vi "Write DIT.vi"(5 "append to file? (default=T)":bool=TRUE, 6 "error in":errorcluster, 7 "String":string, 8 "DIT Key Info":T1, 9 "Filepath In":path) -> (0 "error out":errorcluster, 3 "Filepath Out":path)   [LabVIEW 2013]
doc: "Takes recent Activities text which has already been written to the Activities file and calculates the DIT and then appends the DIT to the Activities file.\n\nWhen this VI is used for images or other non-text file, it creates a new file with just the DIT in the attachment file. The file created has the same name as the Filepath input. Higher level VIs must determine the filename and extension."
uses:
  User Access Type defs/DIT Key cluster.ctl
  GUI/GUI.lvlib
panel:
  out "DIT":string
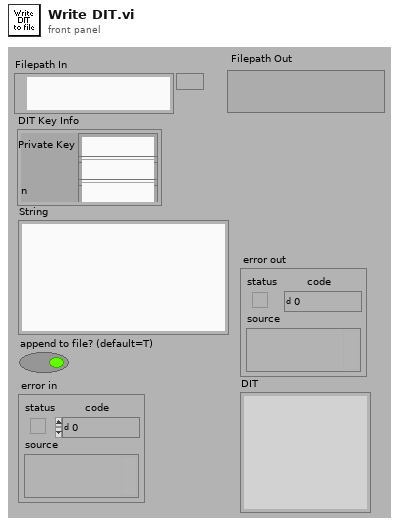
[diagram p1: front panel]
types:
  T1 = typedef "DIT Key cluster.ctl" = cluster{"Private Key":string, "Public Key":string, "n":string}
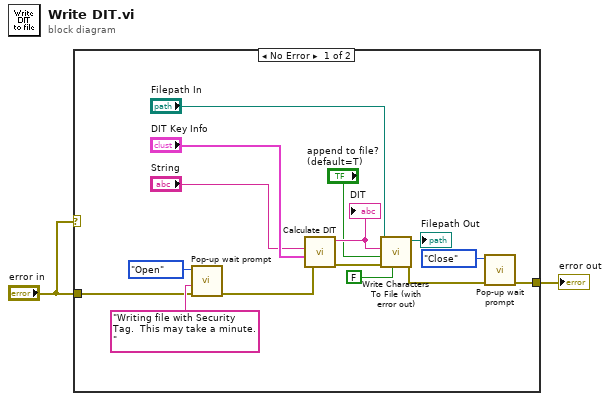
[diagram p0: block diagram]
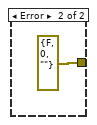
[diagram p2: hidden frame]
diagram:
  n1 = case shown="No Error" "error in" {
    tunnel: "error in" -> [w9 _]
    tunnel: [w5 errorcluster {"status"=FALSE, "code"=0, "source"=""} ("error out")] -> w2
    frame No Error {
      n2 = call "Pop-up wait prompt.vi"("error in (no error)"=w9, "Prompt Text"="Writing file with Security Tag.  This may take a minute.", "Control"=enum16{"Open", "Close", "Status", "No Change"}."Open") -> ("error out"=w8:errorcluster)  [unwired: 1 in, 7 out]
      n3 = call "Calculate DIT.vi"("error in"=w8, "DIT Key Info"="DIT Key Info", "Text without DIT"="String") -> ("error out"=w14:errorcluster, "DIT"=w13:string)  [unwired: 2 in, 1 out]
      "DIT" <- w13
      n4 = call "Write Characters To File (with error out).vi"("advisory dialog? (display:T)"=FALSE, "error in (no error)"=w14, "append to file? (new file:F)"="append to file? (default=T)", "character string"=w13, "file path (dialog if empty)"="Filepath In") -> ("error out"=w6:errorcluster, "new file path (Not A Path if cancelled)"=→"Filepath Out":path)  [unwired: 2 in, 3 out]
      n5 = call "Pop-up wait prompt.vi"("error in (no error)"=w6, "Control"=enum16{"Open", "Close", "Status", "No Change"}."Close") -> ("error out"=w5:errorcluster)  [unwired: 2 in, 7 out]
    }
    frame Error {
    }
  }
  "error out" <- w2
